vi "Colors.vi"() -> ()   [LabVIEW 2013]
panel:
  out "Etiquetas":string[](array[string])
  out "Cluster":T1
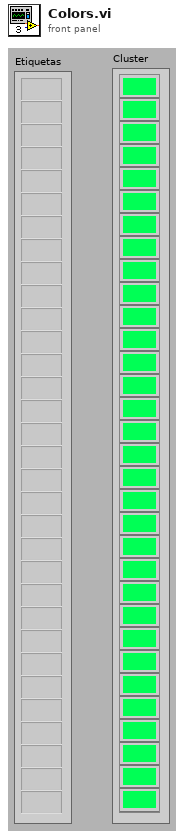
[diagram p1: front panel]
types:
  T1 = cluster{"String":string, "String 2":string, "String 3":string, "String 4":string, "String 5":string, "String 6":string, "String 7":string, "String 8":string, "String 9":string, "String 10":string, "String 11":string, "String 12":string, "String 13":string, "String 14":string, "String 15":string, "String 16":string, "String 17":string, "String 18":string, "String 19":string, "String 20":string, "String 21":string, "String 22":string, "String 23":string, "String 24":string, "String 25":string, "String 26":string, "String 27":string, "String 28":string, "String 29":string, "String 30":string, "String 31":string, "String 32":string}
  T2 = cluster{"Etiquetas[0]":string, "Etiquetas[1]":string, "Etiquetas[2]":string, "Etiquetas[3]":string, "Etiquetas[4]":string, "Etiquetas[5]":string, "Etiquetas[6]":string, "Etiquetas[7]":string, "Etiquetas[8]":string, "Etiquetas[9]":string, "Etiquetas[10]":string, "Etiquetas[11]":string, "Etiquetas[12]":string, "Etiquetas[13]":string, "Etiquetas[14]":string, "Etiquetas[15]":string, "Etiquetas[16]":string, "Etiquetas[17]":string, "Etiquetas[18]":string, "Etiquetas[19]":string, "Etiquetas[20]":string, "Etiquetas[21]":string, "Etiquetas[22]":string, "Etiquetas[23]":string, "Etiquetas[24]":string, "Etiquetas[25]":string, "Etiquetas[26]":string, "Etiquetas[27]":string, "Etiquetas[28]":string, "Etiquetas[29]":string, "Etiquetas[30]":string, "Etiquetas[31]":string}
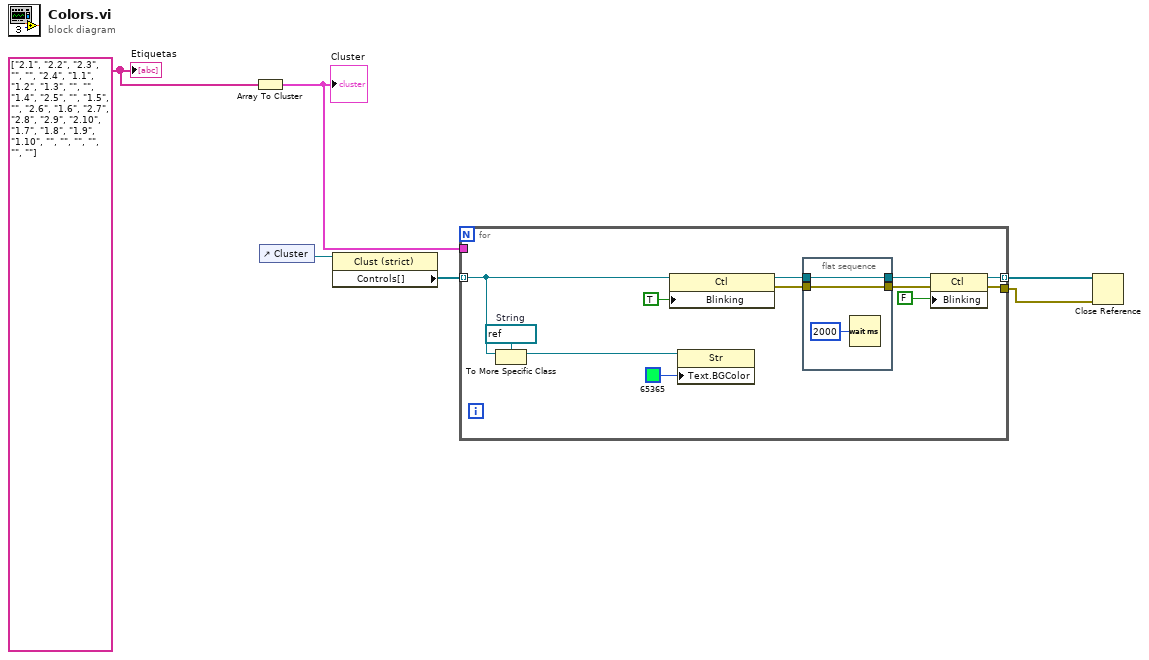
[diagram p0: block diagram]
diagram:
  w6 = string[] ["2.1", "2.2", "2.3", "", "", "2.4", "1.1", "1.2", "1.3", "", "", "1.4", "2.5", "", "1.5", "", "2.6", "1.6", "2.7", "2.8", "2.9", "2.10", "1.7", "1.8", "1.9", "1.10", "", "", "", "", "", ""] ("Etiquetas")
  n1 = Array To Cluster(array=w6) -> (cluster=w4:T2)
  "Cluster" <- w4
  n2 = control-ref of="Cluster"() -> (w3:refnum<vi>)
  n3 = property class="Clust (strict)"(reference=w3) -> ("Controls[]"=w5:refnum<vi>[])  [unwired: 1 in, 2 out]
  n4 = for {
    tunnel: w5 -> [w12] mode=indexing
    tunnel: w4 -> [_]
    tunnel: [w8] -> w2 mode=indexing
    tunnel: [w7] -> w1
    w11 = refnum<vi> refnum  # String
    n5 = To More Specific Class(target class=w11, reference=w12) -> (specific class reference=w10:refnum<vi>)  [unwired: 1 in, 1 out]
    n6 = property class="Ctl"(reference=w12, "Blinking"=TRUE) -> (reference out=w15:refnum<vi>, error out=w14:errorcluster)  [unwired: 1 in]
    n7 = property class="Str"(reference=w10, "Text.BGColor"=u32 65365) -> ()  [unwired: 1 in, 2 out]
    n8 = flat-sequence {
      tunnel: [w20] -> w16
      tunnel: w15 -> [w20]
      tunnel: w14 -> [w19]
      tunnel: [w19] -> w13
      frame #0 {
        n9 = Wait (ms)(milliseconds to wait=u32 2000) -> ()  [unwired: 1 out]
      }
    }
    n10 = property class="Ctl"(reference=w16, error in=w13, "Blinking"=FALSE) -> (reference out=w8:refnum<vi>, error out=w7:errorcluster)
  }
  n11 = Close Reference(reference=w2, error in (no error)=w1) -> ()  [unwired: 1 out]
  "Etiquetas" <- w6
